vi "VirtualPowerPlantWithModelBasedFaultDetection.vi"() -> ()   [LabVIEW 2017, in "HMILibrary.lvlib"]
uses:
  HMILibrary.lvlib
  <vilib>/Platform/TimedLoop/XDataNode/timing_clust.ctl
  <vilib>/Platform/TimedLoop/XDataNode/nitl_modes.ctl
  <vilib>/Platform/TimedLoop/XDataNode/wakeup.ctl
  <vilib>/Utility/file.llb/Write Delimited Spreadsheet (string).vi
  <vilib>/Utility/file.llb/Write Delimited Spreadsheet (DBL).vi
  <vilib>/platform/TimedLoop/XDataNode/XDataNode.xnode
  <vilib>/express/express arith-compare/Formula/XNode/ExpressFormulaBlockNode.xnode
  <vilib>/Platform/TimedLoop/XDataNode/XDNodeRunTimeDep.lvlib
panel:
  in  "Clear Warnings":bool
  in  "Hold Model Inputs Constant":bool
  in  "Reactor Power":dbl=7500.0
  out "Sensor 4":cluster{"placeholder1":dbl, dbl}(graph)
  out "Sensor 3":cluster{"placeholder1":dbl, dbl}(graph)
  out "Sensor 2":cluster{"placeholder1":dbl, dbl}(graph)
  out "Sensor 1":cluster{"placeholder1":dbl, dbl}(graph)
  in  "dTsamplethreshold":dbl=10.0
  in  "Tsamplethreshold":dbl=3.0
  in  "dTthreshold4":dbl=2.1702
  in  "dTthreshold3":dbl=2.8362
  in  "dTthreshold2":dbl=2.6736
  in  "dTthreshold1":dbl=2.361
  in  "Tthreshold4":dbl=0.4812
  in  "Tthreshold3":dbl=1.6494
  in  "Tthreshold2":dbl=0.5934
  in  "Tthreshold1":dbl=0.588
  in  "Weight of measured values in filter":dbl=0.01
  out "Warnings":string
  in  "stop":bool
  out "Cold Leg Temp":dbl
  out "Primary HX Outlet Temp":dbl
  out "Hot Leg Temp":dbl
  out "color3":u32(colorbox)
  out "Heater Outlet Temp":dbl caption="C"
  out "color4":u32(colorbox)
  out "color2":u32(colorbox)
  in  "Upper Operating Pressure":dbl=6154480.5
  in  "Pump Efficiency":dbl=0.95
  in  "Turbine Efficiency":dbl=0.95
  in  "Pinch Point Temp Difference":dbl=15.0
  in  "Lower Operating Pressure":dbl=7093.0
  in  "Mass Flowrate":dbl=418.0
  in  "Pressure Drop in HX 2nd pass":dbl
  in  "Pressure Drop in HX 1st pass":dbl
  in  "LPT Work Output":dbl=137940000.0
  in  "HPT Work Output":dbl=1000000.0
  in  "LPT Efficiency":dbl=0.8
  in  "HPT Efficiency":dbl=0.8
  in  "Compressor Efficiency":dbl=0.7
  in  "LPT Expansion Ratio":dbl=5.13
  in  "Incoming Air Pressure":dbl=101325.0
  in  "HPT Expansion Ratio":dbl=3.77
  in  "Incoming Air Temp":dbl=298.0
  in  "Compression Ratio":dbl=19.6
  out "h_1":dbl
  out "R_T_1":dbl
  out "R_P_1":dbl
  out "h_6":dbl
  out "R_T_6":dbl
  out "R_P_6":dbl
  out "h_5":dbl
  out "R_T_5":dbl
  out "R_P_5":dbl
  out "h_4":dbl
  out "R_T_4":dbl
  out "R_P_4":dbl
  out "T_6":dbl
  out "P_6":dbl
  out "T_5":dbl
  out "P_5":dbl
  out "T_4":dbl
  out "P_4":dbl
  out "T_3":dbl
  out "P_3":dbl
  out "T_2":dbl
  out "P_2":dbl
  out "T_1":dbl
  out "P_1":dbl
  out "color1":u32(colorbox)
  # "Reactor Loop"
  # "Brayton Cycle"
  # "Rankine Cycle"
  # "ST"
  # "HRSG"
  # "Compressor"
  # "HPT"
  # "LPT"
  # "Reactor"
  # "Primary Heat\nExchanger"
  # "Condenser"
  # "Pump"
  # "Pump"
  # "Temperatures in degrees C"
  # "Temperatures in K\nPressures in Pa"
  # "Temperatures in K\nPressures in Pa"
  # "Developer's Tools"
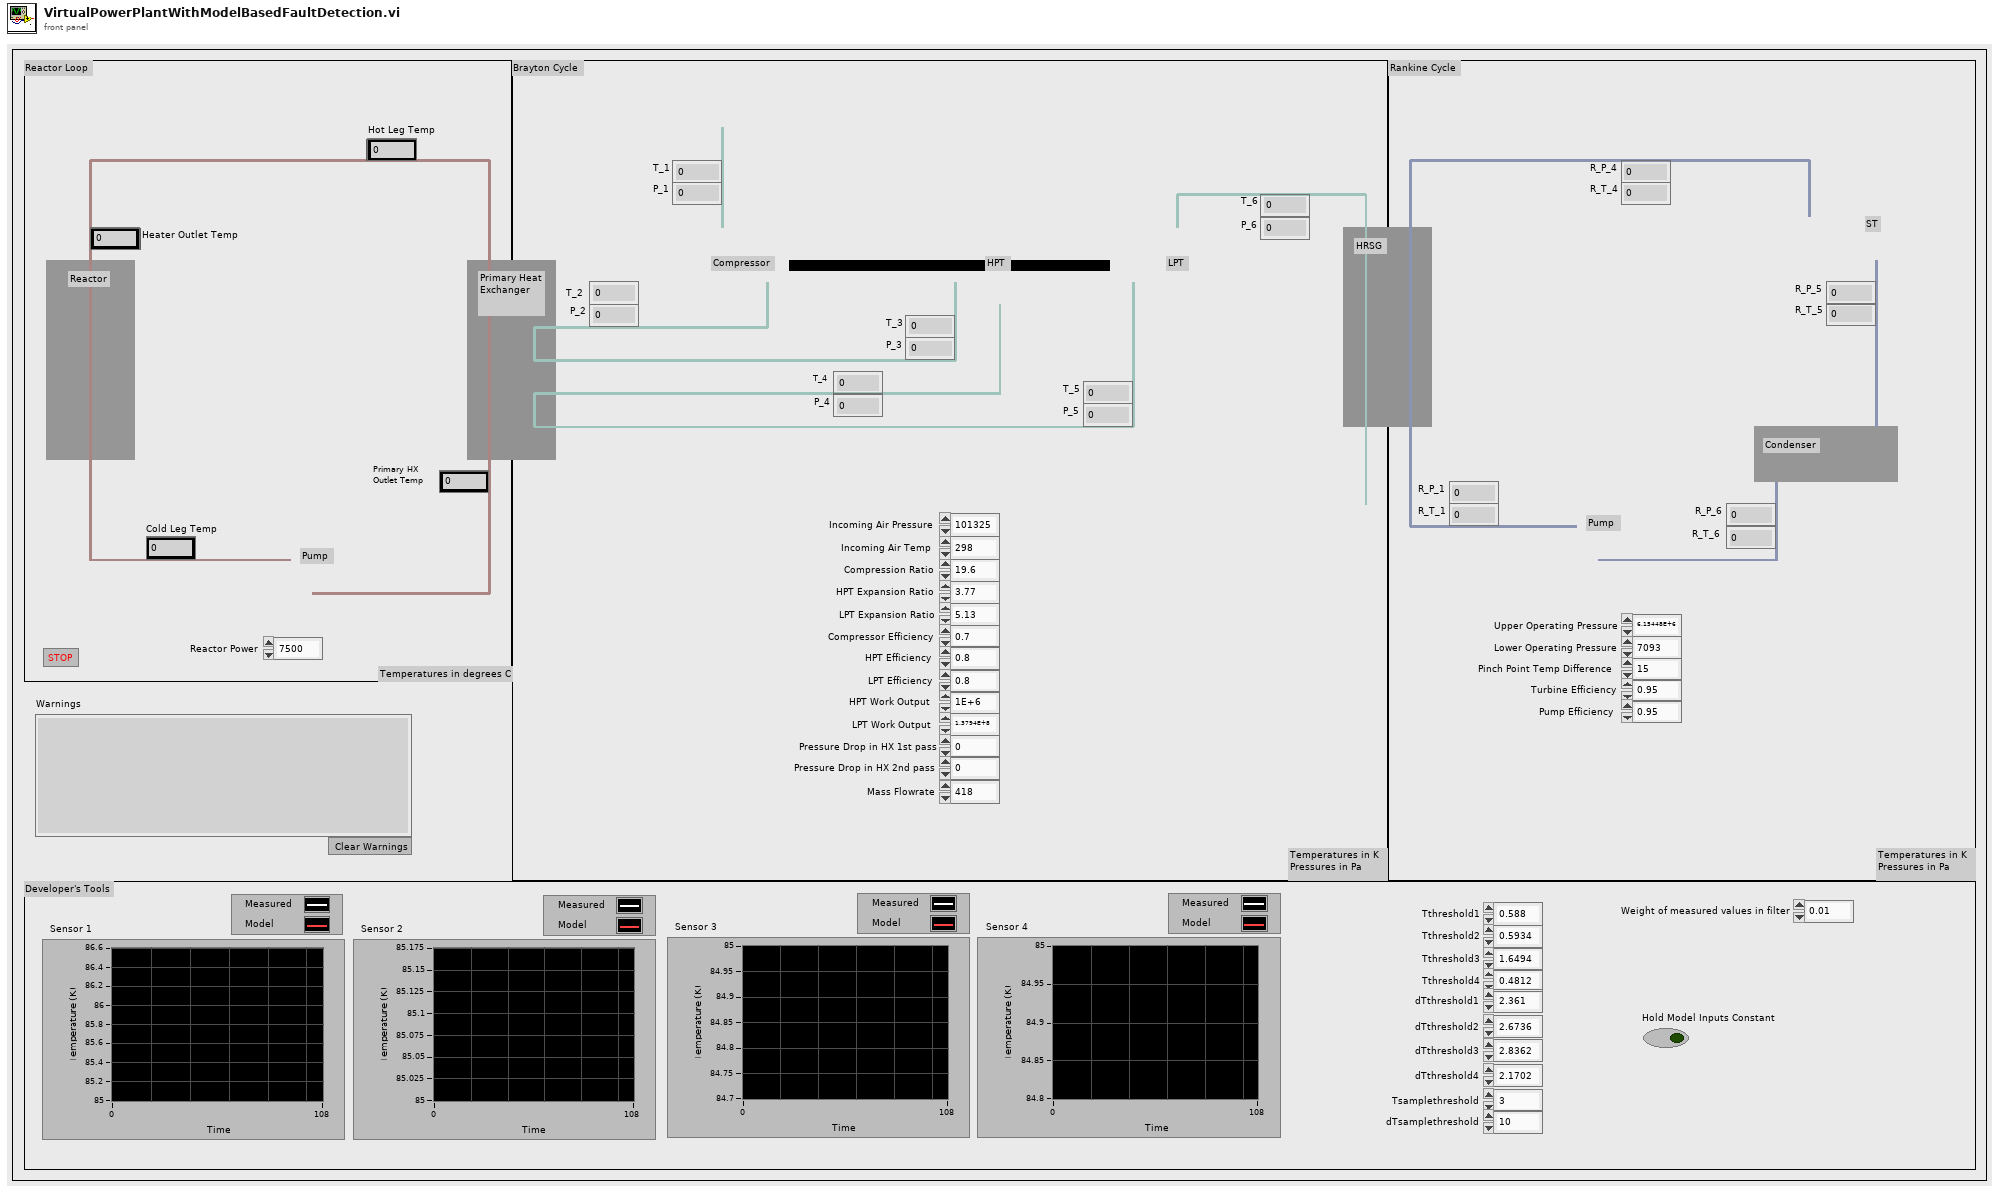
[diagram p1: front panel]
types:
  T1 = typedef "XDNodeRunTimeDep.lvlib/timing_clust.ctl" = cluster{"Expected End [f-1]":u64, "Actual End [f-1]":u64, "Finished Late? [f-1]":bool, "Expected End [i-1]":u64, "Actual End [i-1]":u64, "Finished Late? [i-1]":bool, "Expected Start [i]":u64, "Actual Start [i]":u64, "Expected Start [f]":u64, "Actual Start [f]":u64, "Source Name":string, "Structure Name":string, "Period":i64, "Deadline":i64, "Offset":i64, "Start":i64, "Priority":i32, "Timeout":i32, "Mode":T2, "Wakeup Reason":T3, "Error":errorcluster, "Source Type":string, "Secondary Source Type":string, "Global End Time":u64, "Global Start Time":u64, "Frame Duration":u64, "Iteration Duration":u64, "Assigned CPU":i32, "I/O Scan Engine Mode":u32}
  T2 = typedef "XDNodeRunTimeDep.lvlib/nitl_modes.ctl" = enum32{"No Change", "Process missed periods, maintain original phase", "Discard missed periods, maintain original phase", "Process missed periods, ignore original phase", "Discard missed periods, ignore original phase"}
  T3 = typedef "XDNodeRunTimeDep.lvlib/wakeup.ctl" = enum32{"Normal", "Aborted", "Asynchronous wakeup", "Timing source error", "Timed loop error", "Timeout"}
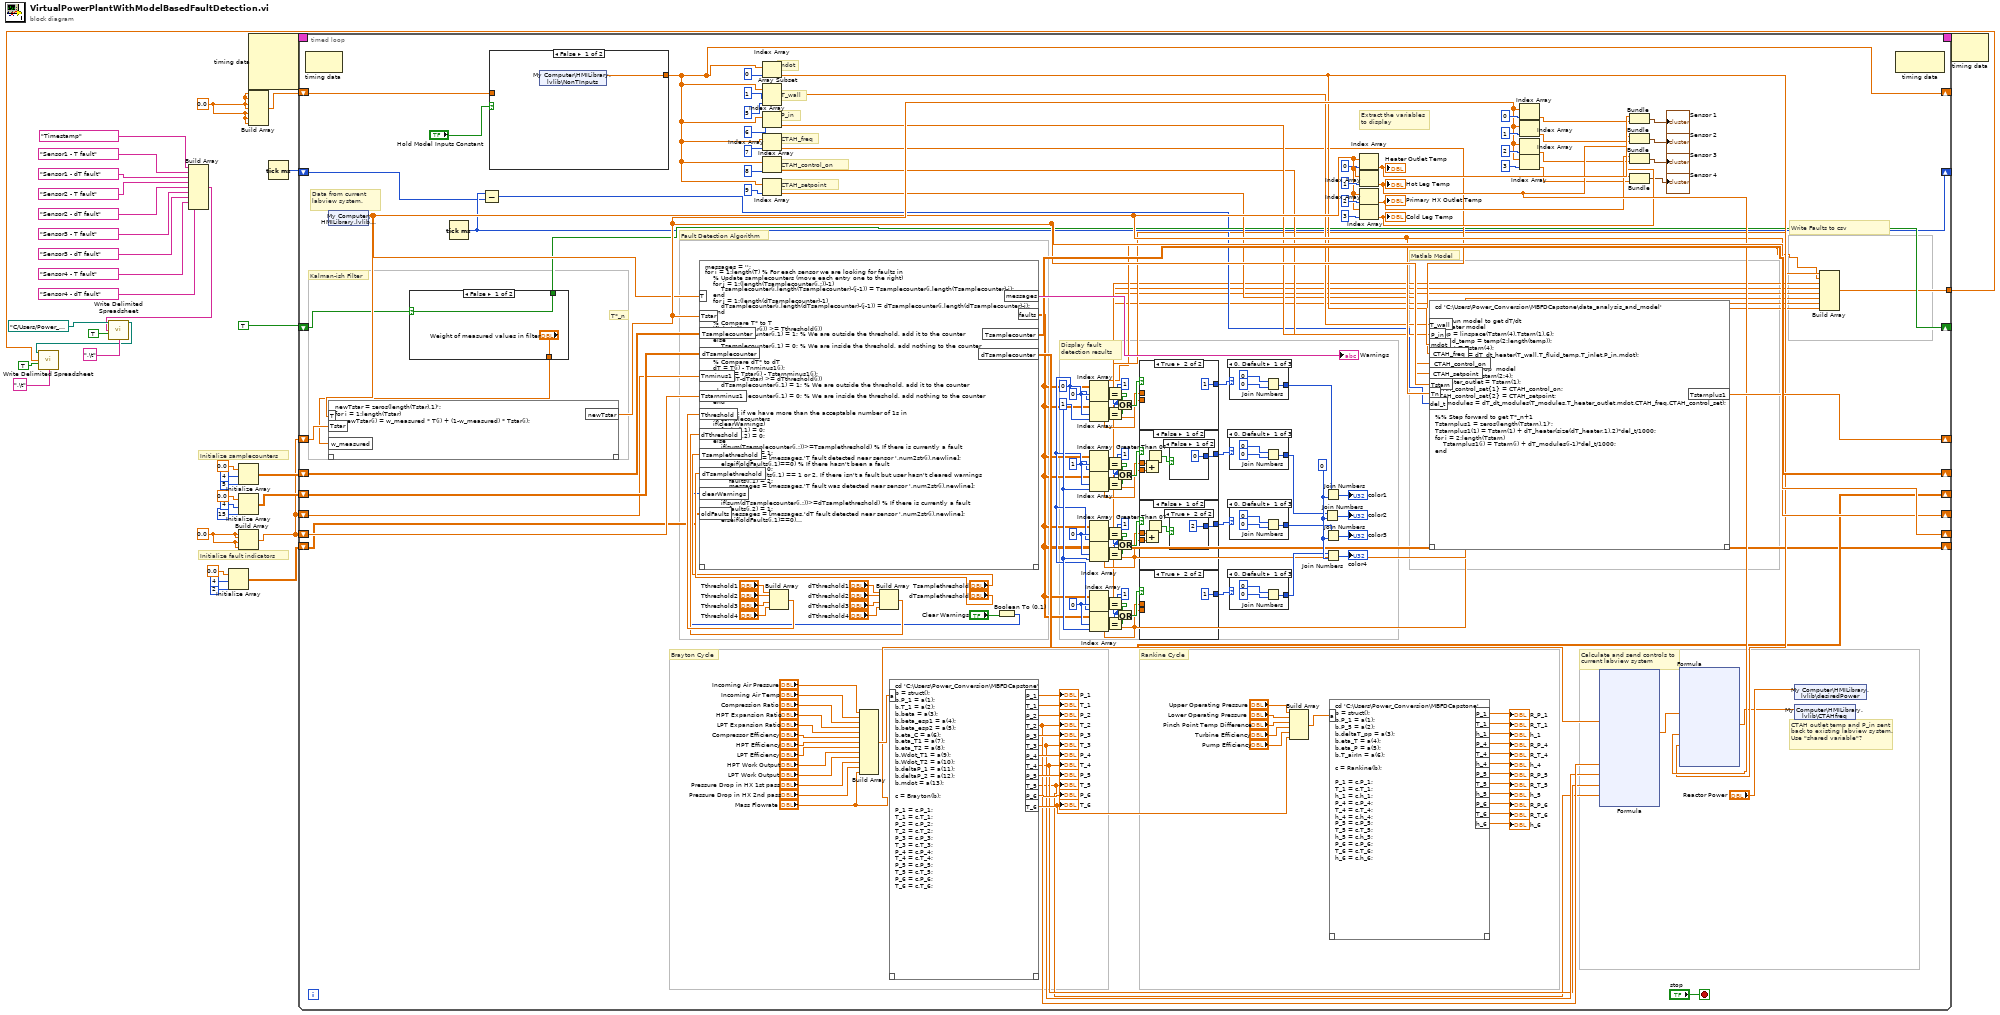
[diagram p0: block diagram]
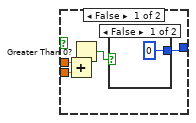
[diagram p2: hidden frame]
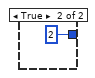
[diagram p3: hidden frame]
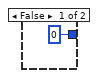
[diagram p4: hidden frame]
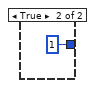
[diagram p5: hidden frame]
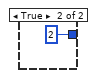
[diagram p6: hidden frame]
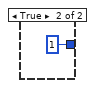
[diagram p7: hidden frame]
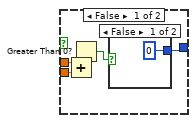
[diagram p8: hidden frame]
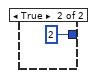
[diagram p9: hidden frame]
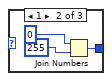
[diagram p10: hidden frame]
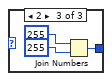
[diagram p11: hidden frame]
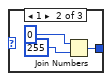
[diagram p12: hidden frame]
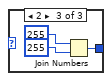
[diagram p13: hidden frame]
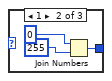
[diagram p14: hidden frame]
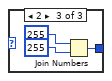
[diagram p15: hidden frame]
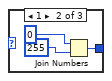
[diagram p16: hidden frame]
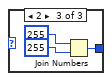
[diagram p17: hidden frame]
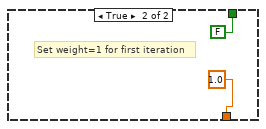
[diagram p18: hidden frame]
diagram:
  w24 = 0.0
  w27 = 0.0
  # "Initialize fault indicators"
  # "Initialize samplecounters"
  n1 = Build Array("Timestamp", "Sensor1 - T fault", "Sensor1 - dT fault", "Sensor2 - T fault", "Sensor2 - dT fault", "Sensor3 - T fault", "Sensor3 - dT fault", "Sensor4 - T fault", "Sensor4 - dT fault") -> (w1:string[])
  n2 = call-poly <vilib>:"Write Delimited Spreadsheet.vi"("file path (dialog if empty)"=path "C:/Users/Power_Conversion/Desktop", "1D data"=w1, "append to file? (new file:F)"=TRUE, "delimiter (\\t)"=",\t" ("delimiter (\\t)")) -> ("new file path (Not A Path if cancelled)"=w13:path)  [unwired: 10 in, 1 out]
  n3 = Initialize Array(0.0, 4, 2) -> (w21:dbl[][])
  n4 = Initialize Array(0.0, 4, 5) -> (w33:dbl[][])
  n5 = Initialize Array(0.0, 4, 15) -> (w32:dbl[][])
  n6 = Build Array(w27, w27, w27, w27) -> (w26:dbl[])
  n7 = node-c288() -> (w37:T1)  [unwired: 4 in]
  n8 = Build Array(w24, w24, w24, w24, w24, w24, w24) -> (w25:dbl[])
  n9 = Tick Count (ms)() -> (millisecond timer value=w18:u32)
  n10 = timed-loop {
    shift-right: [w141] -> _
    shift-left: w26 -> [w140]
    shift-right: [w146] -> _
    shift-left: w33 -> [w145]
    shift-right: [w54] -> _
    shift-left: w32 -> [w144]
    shift-right: [w106] -> _
    shift-left: w26 -> [w143]
    shift-right: [w119] -> _
    shift-left: w26 -> [w142]
    timing: w37 -> [_]
    timing-out: [_] -> w36
    shift-right: [w87] -> _
    shift-left: w25 -> [w91]
    shift-right: [w48] -> _
    shift-left: w21 -> [w88]
    shift-right: [w85] -> _
    shift-left: TRUE -> [w86]
    shift-right: [w83] -> _
    shift-left: w18 -> [w82]
    tunnel: [w40] -> w17
    stop <- "stop" stop-if-true
    w58 = 1
    w59 = 0
    w63 = 1
    w64 = 0
    w69 = 1
    w70 = 1
    w74 = 1
    w53 = 1
    w124 = u8 0
    w52 = 0
    w76 = 0
    # "Write Faults to csv"
    # "CTAH_setpoint"
    # "CTAH_control_on"
    # "CTAH_freq"
    # "P_in"
    # "T_wall"
    # "mdot"
    # "Kalman-ish Filter"
    # "Extract the variables to display"
    # "Data from current labview system."
    # "CTAH outlet temp and P_in sent back to existing labview system. Use \"shared variable\"?"
    # "Calculate and send controls to current labview system"
    # "Display fault detection results"
    # "Fault Detection Algorithm"
    # "T*_n"
    # "Matlab Model"
    # "Rankine Cycle"
    # "Brayton Cycle"
    n11 = node-c288() -> ()  [unwired: 1 in, 1 out]
    n12 = shared-variable "My Computer\\HMILibrary.lvlib\\T_n"() -> (w106:dbl[])  [unwired: 1 in, 1 out]
    n13 = case shown="False" w86 {
      selector: w86 -> [w268 _]
      tunnel: [w268 FALSE] -> w85
      tunnel: ["Weight of measured values in filter" 1.0] -> w84
      frame False {
      }
      frame True {
        # "Set weight=1 for first iteration"
      }
    }
    n14 = script code="newTstar = zeros(length(Tstar),1)';\nfor i = 1:length(Tstar)\n    newTstar(i) = w_measured * T(i) + (1-w_measured) * Tstar(i);\nend"("T"=w106, "Tstar"=w140, "w_measured"=w84) -> ("newTstar"=w119:dbl[])  [unwired: 1 in, 1 out]
    n15 = Tick Count (ms)() -> (millisecond timer value=w83:u32)
    n16 = Subtract(x=w83, y=w82) -> (x-y=w81:u32)
    n17 = case shown="False" "Hold Model Inputs Constant" {
      tunnel: [w271 w272] -> w87
      tunnel: w91 -> [_ w272]
      frame False {
        n18 = shared-variable "My Computer\\HMILibrary.lvlib\\NonTInputs"() -> (w271:dbl[])  [unwired: 1 in, 1 out]
      }
      frame True {
      }
    }
    n19 = Index Array(array=w87, index=0) -> (element=w105:dbl)
    n20 = Array Subset(array=w87, index=1, length=5) -> (w101:dbl[])
    n21 = Index Array(array=w87, index=6) -> (element=w100:dbl)
    n22 = Index Array(array=w87, index=7) -> (element=w97:dbl)
    n23 = Index Array(array=w87, index=8) -> (element=w96:dbl)
    n24 = Index Array(array=w87, index=9) -> (element=w94:dbl)
    n25 = Build Array("Tthreshold1", "Tthreshold2", "Tthreshold3", "Tthreshold4") -> (w135:dbl[])
    n26 = Build Array("Incoming Air Pressure", "Incoming Air Temp", "Compression Ratio", "HPT Expansion Ratio", "LPT Expansion Ratio", "Compressor Efficiency", "HPT Efficiency", "LPT Efficiency", "HPT Work Output", "LPT Work Output", "Pressure Drop in HX 1st pass", "Pressure Drop in HX 2nd pass", "Mass Flowrate") -> (w186:dbl[])
    n27 = Build Array("dTthreshold1", "dTthreshold2", "dTthreshold3", "dTthreshold4") -> (w130:dbl[])
    n28 = script code="cd 'C:\\Users\\Power_Conversion\\MBFDCapstone'\nb = struct();\nb.P_1 = a(1);\nb.T_1 = a(2);\nb.beta = a(3);\nb.beta_esp1 = a(4);\nb.beta_esp2 = a(5);\nb.eta_C = a(6);\nb.eta_T1 = a(7);\nb.eta_T2 = a(8);\nb.Wdot_T1 = a(9);\nb.Wdot_T2 = a(10);\nb.deltaP_1 = a(11);\nb.deltaP_2 = a(12);\nb.mdot = a(13);\n\nc = Brayton(b);\n\nP_1 = c.P_1;\nT_1 = c.T_1;\nP_2 = c.P_2;\nT_2 = c.T_2;\nP_3 = c.P_3;\nT_3 = c.T_3;\nP_4 = c.P_4;\nT_4 = c.T_4;\nP_5 = c.P_5;\nT_5 = c.T_5;\nP_6 = c.P_6;\nT_6 = c.T_6;"("a"=w186) -> ("P_1"=→"P_1":dbl, "T_1"=→"T_1":dbl, "P_2"=→"P_2":dbl, "T_2"=w151:dbl, "P_3"=→"P_3":dbl, "T_3"=w150:dbl, "P_4"=→"P_4":dbl, "T_4"=w149:dbl, "P_5"=→"P_5":dbl, "T_5"=w148:dbl, "P_6"=→"P_6":dbl, "T_6"=w172:dbl)  [unwired: 1 in, 1 out]
    "T_2" <- w151
    "T_3" <- w150
    "T_4" <- w149
    "T_5" <- w148
    "T_6" <- w172
    n29 = Boolean To (0,1)(Boolean="Clear Warnings") -> (0, 1=w89:i16)
    n30 = script code="messages = '';\nfor i = 1:length(T) % For each sensor we are looking for faults in\n    % Update samplecounters (move each entry one to the right)\n    for j = 1:(length(Tsamplecounter(i,:))-1)\n        Tsamplecounter(i,length(Tsamplecounter)-(j-1)) = Tsamplecounter(i,length(Tsamplecounter)-j);\n    end\n    for j = 1:(length(dTsamplecounter)-1)\n        dTsamplecounter(i,length(dTsamplecounter)-(j-1)) = dTsamplecounter(i,length(dTsamplecounter)-j);\n    end\n    \n    % Compare T* to T\n    if(abs(T(i)-Tstar(i)) >= Tthreshold(i))\n        Tsamplecounter(i,1) = 1; % We are outside the threshold, add it to the counter\n    else\n        Tsamplecounter(i,1) = 0; % We are inside the threshold, add nothing to the counter\n    end\n    \n    % Compare dT* to dT\n    dT = T(i) - Tnminus1(i);\n    dTstar = Tstar(i) - Tstarnminus1(i);\n    if(abs(dT-dTstar) >= dTthreshold(i))\n        dTsamplecounter(i,1) = 1; % We are outside the threshold, add it to the counter\n    else\n        dTsamplecounter(i,1) = 0; % We are inside the threshold, add nothing to the counter\n    end\n    \n    % Check if we have more than the acceptable number of 1s in\n    % samplecounters\n    if(clearWarnings)\n        faults(i,1) = 0;\n        faults(i,2) = 0;\n    else\n        if(sum(Tsamplecounter(i,:))>=Tsamplethreshold) % If there is currently a fault\n            faults(i,1) = 1;\n            messages = [messages,'T fault detected near sensor ',num2str(i),newline];\n        elseif(oldFaults(i,1)==0) % If there hasn't been a fault\n            faults(i,1) = 0;\n        else % oldFaults(i,1) == 1 or 2, If there isn't a fault but user hasn't cleared warnings\n            faults(i,1) = 2;\n            messages = [messages,'T fault was detected near sensor ',num2str(i),newline];\n        end\n        \n        if(sum(dTsamplecounter(i,:))>=dTsamplethreshold) % If there is currently a fault\n            faults(i,2) = 1;\n            messages = [messages,'dT fault detected near sensor ',num2str(i),newline];\n        elseif(oldFaults(i,1)==0) % If there hasn't been a fault\n            faults(i,2) = 0;\n        else % oldFaults(i,1) == 1 or 2, If there isn't a fault but user hasn't cleared warnings\n            faults(i,2) = 2;\n            messages = [messages,'dT fault was detected near sensor ',num2str(i),newline];\n        end\n    end\nend"("T"=w106, "Tstar"=w119, "Tsamplecounter"=w145, "dTsamplecounter"=w144, "Tnminus1"=w143, "Tstarnminus1"=w142, "Tthreshold"=w135, "dTthreshold"=w130, "Tsamplethreshold"="Tsamplethreshold", "dTsamplethreshold"="dTsamplethreshold", "clearWarnings"=w89, "oldFaults"=w88) -> ("faults"=w48:dbl[][], "messages"=→"Warnings":string, "Tsamplecounter"=w146:dbl[][], "dTsamplecounter"=w54:dbl[][])  [unwired: 1 in, 1 out]
    n31 = Index Array(array=w48, index (row)=w76, index (col)=w52) -> (element=w49:dbl)
    n32 = Index Array(array=w48, index (row)=w76, index (col)=w53) -> (element=w47:dbl)
    n33 = Index Array(array=w48, index (row)=w70, index (col)=w52) -> (element=w46:dbl)
    n34 = Index Array(array=w48, index (row)=w70, index (col)=w53) -> (element=w45:dbl)
    n35 = Index Array(array=w48, index (row)=w64, index (col)=w52) -> (element=w44:dbl)
    n36 = Index Array(array=w48, index (row)=w64, index (col)=w53) -> (element=w43:dbl)
    n37 = Index Array(array=w48, index (row)=w59, index (col)=w52) -> (element=w42:dbl)
    n38 = Index Array(array=w48, index (row)=w59, index (col)=w53) -> (element=w41:dbl)
    n39 = Equal?(x=w74, y=w49) -> (x = y?=w72:bool)
    n40 = Equal?(x=w74, y=w47) -> (x = y?=w73:bool)
    n41 = Equal?(x=w69, y=w46) -> (x = y?=w67:bool)
    n42 = Equal?(x=w69, y=w45) -> (x = y?=w68:bool)
    n43 = Equal?(x=w63, y=w44) -> (x = y?=w61:bool)
    n44 = Equal?(x=w63, y=w43) -> (x = y?=w62:bool)
    n45 = Equal?(x=w58, y=w42) -> (x = y?=w56:bool)
    n46 = Equal?(x=w58, y=w41) -> (x = y?=w57:bool)
    n47 = Or(x=w72, y=w73) -> (x .or. y?=w71:bool)
    n48 = Or(x=w67, y=w68) -> (x .or. y?=w66:bool)
    n49 = Or(x=w61, y=w62) -> (x .or. y?=w60:bool)
    n50 = Or(x=w56, y=w57) -> (x .or. y?=w55:bool)
    n51 = case shown="True" w71 {
      tunnel: [w223 1] -> w75
      tunnel: w49 -> [w227 _]
      tunnel: w47 -> [w226 _]
      frame False {
        n52 = Add(x=w227, y=w226) -> (x+y=w224:dbl)
        n53 = Greater Than 0?(x=w224) -> (x > 0?=w225:bool)
        n54 = case shown="False" w225 {
          tunnel: [0 2] -> w223
          frame False {
          }
          frame True {
          }
        }
      }
      frame True {
      }
    }
    n55 = case shown="False" w66 {
      tunnel: [w215 1] -> w65
      tunnel: w46 -> [w219 _]
      tunnel: w45 -> [w218 _]
      frame False {
        n56 = Add(x=w219, y=w218) -> (x+y=w216:dbl)
        n57 = Greater Than 0?(x=w216) -> (x > 0?=w217:bool)
        n58 = case shown="False" w217 {
          tunnel: [0 2] -> w215
          frame False {
          }
          frame True {
          }
        }
      }
      frame True {
      }
    }
    n59 = case shown="False" w60 {
      tunnel: [w207 1] -> w50
      tunnel: w44 -> [w211 _]
      tunnel: w43 -> [w210 _]
      frame False {
        n60 = Add(x=w211, y=w210) -> (x+y=w208:dbl)
        n61 = Greater Than 0?(x=w208) -> (x > 0?=w209:bool)
        n62 = case shown="True" w209 {
          tunnel: [0 2] -> w207
          frame False {
          }
          frame True {
          }
        }
      }
      frame True {
      }
    }
    n63 = case shown="True" w55 {
      tunnel: [w199 1] -> w51
      tunnel: w42 -> [w203 _]
      tunnel: w41 -> [w202 _]
      frame False {
        n64 = Add(x=w203, y=w202) -> (x+y=w200:dbl)
        n65 = Greater Than 0?(x=w200) -> (x > 0?=w201:bool)
        n66 = case shown="False" w201 {
          tunnel: [0 2] -> w199
          frame False {
          }
          frame True {
          }
        }
      }
      frame True {
      }
    }
    n67 = case shown="0, Default" w75 {
      tunnel: [w258 w261 w264] -> w80
      frame 0, Default {
        n68 = Join Numbers(hi=u8 0, lo=u8 0) -> ((hi.lo)=w258:u16)
      }
      frame 1 {
        n69 = Join Numbers(hi=u8 0, lo=u8 255) -> ((hi.lo)=w261:u16)
      }
      frame 2 {
        n70 = Join Numbers(hi=u8 255, lo=u8 255) -> ((hi.lo)=w264:u16)
      }
    }
    n71 = case shown="0, Default" w65 {
      tunnel: [w249 w252 w255] -> w79
      frame 0, Default {
        n72 = Join Numbers(hi=u8 0, lo=u8 0) -> ((hi.lo)=w249:u16)
      }
      frame 1 {
        n73 = Join Numbers(hi=u8 0, lo=u8 255) -> ((hi.lo)=w252:u16)
      }
      frame 2 {
        n74 = Join Numbers(hi=u8 255, lo=u8 255) -> ((hi.lo)=w255:u16)
      }
    }
    n75 = case shown="0, Default" w50 {
      tunnel: [w240 w243 w246] -> w78
      frame 0, Default {
        n76 = Join Numbers(hi=u8 0, lo=u8 0) -> ((hi.lo)=w240:u16)
      }
      frame 1 {
        n77 = Join Numbers(hi=u8 0, lo=u8 255) -> ((hi.lo)=w243:u16)
      }
      frame 2 {
        n78 = Join Numbers(hi=u8 255, lo=u8 255) -> ((hi.lo)=w246:u16)
      }
    }
    n79 = case shown="0, Default" w51 {
      tunnel: [w231 w234 w237] -> w77
      frame 0, Default {
        n80 = Join Numbers(hi=u8 0, lo=u8 0) -> ((hi.lo)=w231:u16)
      }
      frame 1 {
        n81 = Join Numbers(hi=u8 0, lo=u8 255) -> ((hi.lo)=w234:u16)
      }
      frame 2 {
        n82 = Join Numbers(hi=u8 255, lo=u8 255) -> ((hi.lo)=w237:u16)
      }
    }
    n83 = Build Array("Upper Operating Pressure", "Lower Operating Pressure", "Pinch Point Temp Difference", "Turbine Efficiency", "Pump Efficiency", w172) -> (w173:dbl[])
    n84 = Join Numbers(hi=w79, lo=w124) -> ((hi.lo)=→"color2":u32)
    n85 = Join Numbers(hi=w80, lo=w124) -> ((hi.lo)=→"color1":u32)
    n86 = Join Numbers(hi=w78, lo=w124) -> ((hi.lo)=→"color3":u32)
    n87 = Join Numbers(hi=w77, lo=w124) -> ((hi.lo)=→"color4":u32)
    n88 = script code="cd 'C:\\Users\\Power_Conversion\\MBFDCapstone'\nb = struct();\nb.P_1 = a(1);\nb.P_5 = a(2);\nb.deltaT_pp = a(3);\nb.eta_T = a(4);\nb.eta_P = a(5);\nb.T_airIn = a(6);\n\nc = Rankine(b);\n\nP_1 = c.P_1;\nT_1 = c.T_1;\nh_1 = c.h_1;\nP_4 = c.P_4;\nT_4 = c.T_4;\nh_4 = c.h_4;\nP_5 = c.P_5;\nT_5 = c.T_5;\nh_5 = c.h_5;\nP_6 = c.P_6;\nT_6 = c.T_6;\nh_6 = c.h_6;"("a"=w173) -> ("P_1"=→"R_P_1":dbl, "T_1"=→"R_T_1":dbl, "h_1"=→"h_1":dbl, "P_4"=→"R_P_4":dbl, "T_4"=→"R_T_4":dbl, "h_4"=→"h_4":dbl, "P_5"=→"R_P_5":dbl, "T_5"=→"R_T_5":dbl, "h_5"=→"h_5":dbl, "P_6"=→"R_P_6":dbl, "T_6"=→"R_T_6":dbl, "h_6"=→"h_6":dbl)  [unwired: 1 in, 1 out]
    n89 = Index Array(array=w106, index=0) -> (element=w118:dbl)
    "Heater Outlet Temp" <- w118
    n90 = Index Array(array=w106, index=1) -> (element=w117:dbl)
    "Hot Leg Temp" <- w117
    n91 = Index Array(array=w106, index=2) -> (element=w116:dbl)
    "Primary HX Outlet Temp" <- w116
    n92 = Index Array(array=w106, index=3) -> (element=w115:dbl)
    "Cold Leg Temp" <- w115
    n93 = script code="cd 'C:\\Users\\Power_Conversion\\MBFDCapstone\\data_analysis_and_model'\n\n%% Run model to get dT/dt\n% Heater model\ntemp = linspace(Tstarn(4),Tstarn(1),6);\nT_fluid_temp = temp(2:length(temp));\nT_inlet = Tstarn(4);\ndT_heater = dT_dt_heater(T_wall,T_fluid_temp,T_inlet,P_in,mdot);\n\n% Rest of the loop  model\nT_modules = Tstarn(2:4);\nT_heater_outlet = Tstarn(1);\nCTAH_control_set{1} = CTAH_control_on;\nCTAH_control_set{2} = CTAH_setpoint;\ndT_modules = dT_dt_modules(T_modules,T_heater_outlet,mdot,CTAH_freq,CTAH_control_set);\n\n%% Step forward to get T*_n+1\nTstarnplus1 = zeros(length(Tstarn),1)';\nTstarnplus1(1) = Tstarn(1) + dT_heater(size(dT_heater,1),2)*del_t/1000;\nfor i = 2:length(Tstarn)\n    Tstarnplus1(i) = Tstarn(i) + dT_modules(i-1)*del_t/1000;\nend"("Tstarn"=w119, "T_wall"=w101, "P_in"=w100, "mdot"=w105, "Tn"=w106, "CTAH_freq"=w97, "CTAH_control_on"=w96, "CTAH_setpoint"=w94, "del_t"=w81) -> ("Tstarnplus1"=w141:dbl[])  [unwired: 1 in, 1 out]
    n94 = Index Array(array=w119, index=0) -> (element=w114:dbl)
    n95 = Index Array(array=w119, index=1) -> (element=w113:dbl)
    n96 = Index Array(array=w119, index=2) -> (element=w112:dbl)
    n97 = Index Array(array=w119, index=3) -> (element=w111:dbl)
    n98 = xnode "Formula"("mdot"="Mass Flowrate", "T2"=w151, "T3"=w150, "T4"=w149, "T5"=w148) -> ("Result"=w147:dbl)  [unwired: 1 in, 1 out]
    n99 = Bundle("Numeric"=w118, w114) -> (→"Sensor 1":cluster{"Numeric":dbl, dbl})  [unwired: 1 in]
    n100 = Bundle("Numeric"=w117, w113) -> (→"Sensor 2":cluster{"Numeric":dbl, dbl})  [unwired: 1 in]
    n101 = Bundle("Numeric"=w116, w112) -> (→"Sensor 3":cluster{"Numeric":dbl, dbl})  [unwired: 1 in]
    n102 = Bundle("Numeric"=w115, w111) -> (→"Sensor 4":cluster{"Numeric":dbl, dbl})  [unwired: 1 in]
    n103 = xnode "Formula"("Pout"=w147, "Tin"=w117, "mdot"=w105) -> ("Result"=w38:dbl)  [unwired: 2 in, 1 out]
    n104 = shared-variable "My Computer\\HMILibrary.lvlib\\desiredPower"("Reactor Power") -> ()  [unwired: 1 in, 1 out]
    n105 = shared-variable "My Computer\\HMILibrary.lvlib\\CTAHfreq"(w38) -> ()  [unwired: 1 in, 1 out]
    n106 = Build Array(w49, w47, w46, w45, w44, w43, w42, w41) -> (w40:dbl[])
    n107 = node-c288() -> ()  [unwired: 1 in, 1 out]
  }
  n108 = call-poly <vilib>:"Write Delimited Spreadsheet.vi"("file path (dialog if empty)"=w13, "1D data"=w17, "append to file? (new file:F)"=TRUE, "delimiter (\\t)"=",\t" ("delimiter (\\t)")) -> ()  [unwired: 10 in, 2 out]
  n109 = node-c288(w36) -> ()  [unwired: 1 out]
